vi "addLandmark.vi"(8 "P":dbl[][](array[numeric]), 9 "dX":dbl[](array[numeric]), 10 "X":dbl[](array[numeric]), 11 "newLandmark":dbl[](array[numeric])) -> (2 "P out":dbl[][](array[numeric]), 3 "X out":dbl[](array[numeric]))   [LabVIEW 2009, in "LV_SLAM.lvlib"]
uses:
  LV_SLAM.lvlib
  <vilib>/Analysis/Matrix/Numeric/Add/Add - RM,RM.vi
  <vilib>/Analysis/Matrix/Numeric/Multiply/Multiply - RM,RM.vi
  <vilib>/Analysis/Matrix/Numeric/Conversions/Array To Matrix - RA2.vi
  <vilib>/Analysis/Matrix/NI_Matrix.lvlib
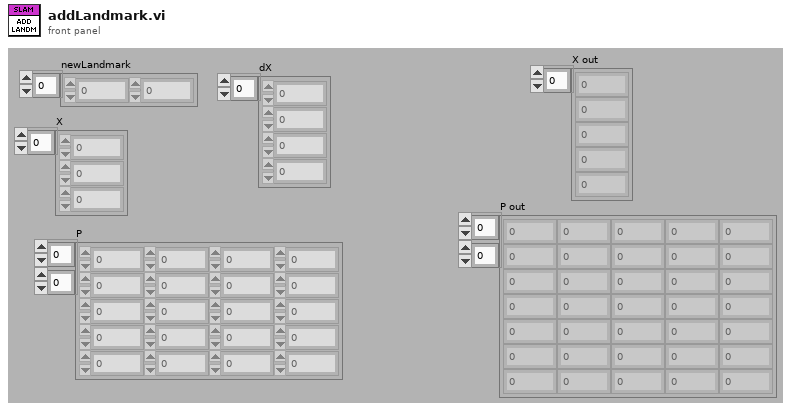
[diagram p1: front panel]
types:
  T1 = typedef "NI_Matrix.lvlib/RealMatrix.ctl" = dbl[][]
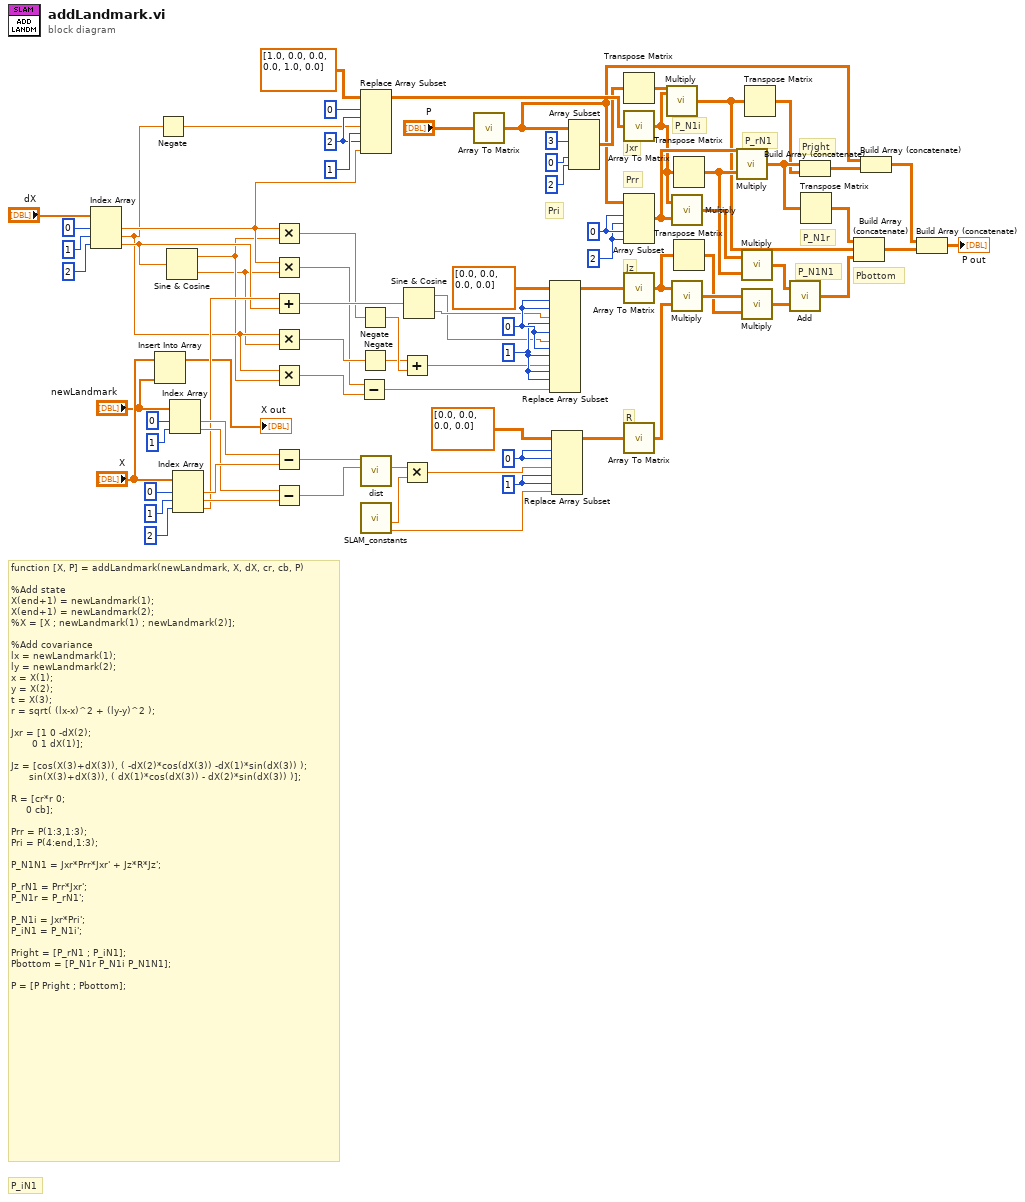
[diagram p0: block diagram]
diagram:
  w30 = 2 ("row N")
  w31 = 0 ("row 1")
  w37 = 1 ("index (row)")
  w38 = 0 ("index (row)")
  w55 = 1 ("index (row)")
  w56 = 0 ("index (row)")
  w61 = 2 ("disabled index (col)")
  # "Pbottom"
  # "Pright"
  # "P_iN1"
  # "P_N1i"
  # "P_N1r"
  # "P_rN1"
  # "P_N1N1"
  # "Pri"
  # "Prr"
  # "R"
  # "Jz"
  # "Jxr"
  # "function [X, P] = addLandmark(newLandmark, X, dX, cr, cb, P)\n\n%Add state\nX(end+1) = newLandmark(1);\nX(end+1) = newLandmark(2);\n%X = [X ; newLandmark(1) ; newLandmark(2)];\n\n%Add covariance\nlx = newLandmark(1);\nly = newLandmark(2);\nx = X(1);\ny = X(2);\nt = X(3);\nr = sqrt( (lx-x)^2 + (ly-y)^2 );\n\nJxr = [1 0 -dX(2);\n       0 1 dX(1)];\n\nJz = [cos(X(3)+dX(3)), ( -dX(2)*cos(dX(3)) -dX(1)*sin(dX(3)) );\n      sin(X(3)+dX(3)), ( dX(1)*cos(dX(3)) - dX(2)*sin(dX(3)) )];\n\nR = [cr*r 0;\n     0 cb];\n\nPrr = P(1:3,1:3);\nPri = P(4:end,1:3);\n\nP_N1N1 = Jxr*Prr*Jxr' + Jz*R*Jz';\n\nP_rN1 = Prr*Jxr';\nP_N1r = P_rN1';\n\nP_N1i = Jxr*Pri';\nP_iN1 = P_N1i';\n\nPright = [P_rN1 ; P_iN1];\nPbottom = [P_N1r P_N1i P_N1N1];\n\nP = [P Pright ; Pbottom];"
  n1 = Index Array(array="dX", index #1=0 ("index"), index #2=1 ("index"), index #3=2 ("index")) -> (element #1=w51:dbl, element #2=w50:dbl, element #3=w52:dbl)
  n2 = Insert Into Array(array="X", new element="newLandmark") -> (→"X out":dbl[])  [unwired: 1 in]
  n3 = Negate(x=w50) -> (-x=w60:dbl)
  n4 = Sine & Cosine(0:w52) -> (1:w49:dbl, 2:w48:dbl)
  n5 = Index Array(array="newLandmark", index #1=0 ("index"), index #2=1 ("index")) -> (element #1=w74:dbl, element #2=w72:dbl)
  n6 = Index Array(array="X", index #1=0 ("index"), index #2=1 ("index"), index #3=2 ("index")) -> (element #1=w73:dbl, element #2=w71:dbl, element #3=w59:dbl)
  n7 = Multiply(x=w51, y=w49) -> (x*y=w46:dbl)
  n8 = Multiply(x=w51, y=w48) -> (x*y=w42:dbl)
  n9 = Add(x=w59, y=w52) -> (x+y=w58:dbl)
  n10 = Multiply(x=w50, y=w48) -> (x*y=w47:dbl)
  n11 = Multiply(x=w50, y=w49) -> (x*y=w41:dbl)
  n12 = Subtract(x=w74, y=w73) -> (x-y=w70:dbl)
  n13 = Subtract(x=w72, y=w71) -> (x-y=w69:dbl)
  n14 = Subtract(x=w42, y=w41) -> (x-y=w40:dbl)
  n15 = Negate(x=w46) -> (-x=w45:dbl)
  n16 = Negate(x=w47) -> (-x=w44:dbl)
  n17 = Replace Array Subset(array=dbl[][] [[1.0, 0.0, 0.0], [0.0, 1.0, 0.0]] ("P"), new element #1=w60, index (row) #1=0 ("index (row)"), index (col) #1=w61, new element #2=w51, index (row) #2=1 ("index (row)"), index (col) #2=w61) -> (w26:dbl[][])
  n18 = call "dist.vi"("y"=w69, "x"=w70) -> ("d"=w36:dbl)  [unwired: 9 in]
  n19 = call "SLAM_constants.vi"() -> ("cb"=w33:dbl, "cr"=w35:dbl)  [unwired: 7 in, 3 out]
  n20 = Add(x=w44, y=w45) -> (x+y=w43:dbl)
  n21 = Multiply(x=w36, y=w35) -> (x*y=w34:dbl)
  n22 = Sine & Cosine(0:w58) -> (1:w53:dbl, 2:w54:dbl)
  n23 = call-poly <vilib>:"Array To Matrix.vi"("Real 2D Array"="P") -> ("Real Matrix"=w6:T1)
  n24 = Replace Array Subset(array=dbl[][] [[0.0, 0.0], [0.0, 0.0]] ("P"), new element #1=w54, index (row) #1=w56, index (col) #1=w56, new element #2=w53, index (row) #2=w55, index (col) #2=w56, new element #3=w43, index (row) #3=w56, index (col) #3=w55, new element #4=w40, index (row) #4=w55, index (col) #4=w55) -> (w25:dbl[][])
  n25 = Replace Array Subset(array=dbl[][] [[0.0, 0.0], [0.0, 0.0]] ("P"), new element #1=w34, index (row) #1=w38, index (col) #1=w38, new element #2=w33, index (row) #2=w37, index (col) #2=w37) -> (w24:dbl[][])
  n26 = Array Subset(array=w6, index (row)=3 ("row 1"), index (col)=0 ("row 1"), length (col)=2 ("row N")) -> (w14:T1)  [unwired: 1 in]
  n27 = Transpose Matrix(1:w14) -> (0:w12:T1)
  n28 = call-poly <vilib>:"Array To Matrix.vi"("Real 2D Array"=w26) -> ("Real Matrix"=w13:T1)
  n29 = Array Subset(array=w6, index (row)=w31, length (row)=w30, index (col)=w31, length (col)=w30) -> (w16:T1)
  n30 = call-poly <vilib>:"Array To Matrix.vi"("Real 2D Array"=w25) -> ("Real Matrix"=w22:T1)
  n31 = call-poly <vilib>:"Array To Matrix.vi"("Real 2D Array"=w24) -> ("Real Matrix"=w21:T1)
  n32 = call-poly <vilib>:"Multiply.vi"("Real Matrix B"=w12, "Real Matrix A"=w13) -> ("A * B"=w8:T1)
  n33 = call-poly <vilib>:"Multiply.vi"("Real Matrix B"=w16, "Real Matrix A"=w13) -> ("A * B"=w23:T1)
  n34 = call-poly <vilib>:"Multiply.vi"("Real Matrix B"=w21, "Real Matrix A"=w22) -> ("A * B"=w20:T1)
  n35 = Transpose Matrix(1:w13) -> (0:w15:T1)
  n36 = Transpose Matrix(1:w22) -> (0:w19:T1)
  n37 = call-poly <vilib>:"Multiply.vi"("Real Matrix B"=w15, "Real Matrix A"=w16) -> ("A * B"=w11:T1)
  n38 = call-poly <vilib>:"Multiply.vi"("Real Matrix B"=w15, "Real Matrix A"=w23) -> ("A * B"=w18:T1)
  n39 = call-poly <vilib>:"Multiply.vi"("Real Matrix B"=w19, "Real Matrix A"=w20) -> ("A * B"=w17:T1)
  n40 = Transpose Matrix(1:w8) -> (0:w10:T1)
  n41 = call-poly <vilib>:"Add.vi"("Real Matrix B"=w17, "Real Matrix A"=w18) -> ("A + B"=w7:T1)
  n42 = Build Array (concatenate)(w11, w10) -> (w5:T1)
  n43 = Transpose Matrix(1:w11) -> (0:w9:T1)
  n44 = Build Array (concatenate)(w9, w8, w7) -> (w3:T1)
  n45 = Build Array (concatenate)(w6, w5) -> (w4:T1)
  n46 = Build Array (concatenate)(w4, w3) -> (→"P out":T1)
